vi "solar_voy_def Variant Get TCP.vi"(8 "error in (no error)":errorcluster, 11 "Variant":variant) -> (0 "error out":errorcluster, 2 "LabVIEW Flattened Value":string[](array[string]), 3 "LabVIEW Values":variant[](array[variant]))   [LabVIEW 2018]
doc: "This unpacks a variant into an array of variants. Paths are converted into strings."
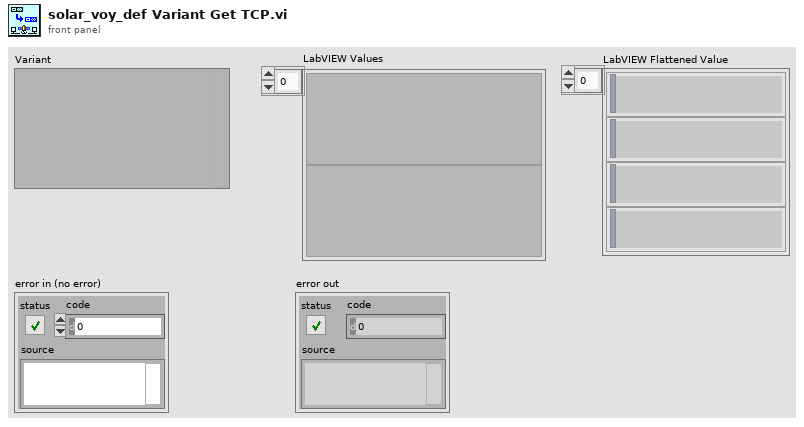
[diagram p1: front panel]
types:
  T1 = typedef "solar_type Item Type.ctl" = enum16{"NULL", "UNKNOWN", "CLUSTER", "I8", "I16", "I32", "I64", "U8", "U16", "U32", "U64", "U8_ENUM", "U16_ENUM", "U32_ENUM", "SGL", "DBL", "BOOLEAN", "STRING", "PATH", "VISA", "TAG", "TIME", "I8_1D", "I16_1D", "I32_1D", "I64_1D", "U8_1D", "U16_1D", "U32_1D", "U64_1D", "U8_ENUM_1D", "U16_ENUM_1D", "U32_ENUM_1D", "SGL_1D", "DBL_1D", "BOOLEAN_1D", "STRING_1D", "PATH_1D", "VISA_1D", "TAG_1D", "TIME_1D", "I8_2D", "I16_2D", "I32_2D", "I64_2D", "U8_2D", "U16_2D", "U32_2D", "U64_2D", "U8_ENUM_2D", "U16_ENUM_2D", "U32_ENUM_2D", "SGL_2D", "DBL_2D", "BOOLEAN_2D", "STRING_2D", "PATH_2D", "VISA_2D", "TAG_2D", "TIME_2D"}
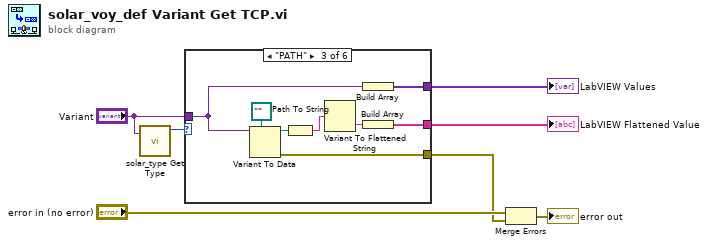
[diagram p0: block diagram]
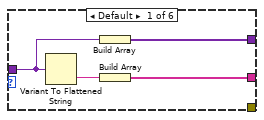
[diagram p2: hidden frame]
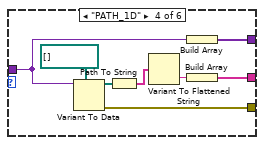
[diagram p4: hidden frame]
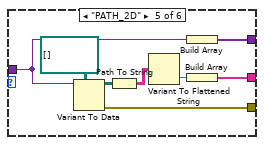
[diagram p5: hidden frame]
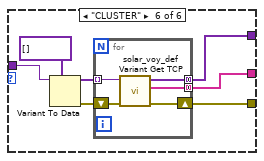
[diagram p6: hidden frame]
diagram:
  n1 = call "solar_type Get Type.vi"("Variant"="Variant") -> ("Type"=w2:T1)  [unwired: 4 in, 2 out]
  n2 = case shown="\"PATH\"" w2 {
    tunnel: "Variant" -> [w9 _ w13 w21 w29 w42]
    tunnel: [w10 _ w14 w22 w30 w39] -> w7
    tunnel: [_ _ w19 w27 w35 w37] -> w5
    tunnel: [w8 _ w12 w20 w28 w36] -> w1
    frame Default {
      n3 = Variant To Flattened String(Variant=w9) -> (data string=w11:string)  [unwired: 1 out]
      n4 = Build Array(w9) -> (w8:variant[])
      n5 = Build Array(w11) -> (w10:string[])
    }
    frame "NULL" {
    }
    frame "PATH" {
      n6 = Variant To Data(type=path "", Variant=w13) -> (data=w17:path, error out=w19:errorcluster)  [unwired: 1 in]
      n7 = Path To String(path=w17) -> (string=w16:string)
      n8 = Variant To Flattened String(Variant=w16) -> (data string=w15:string)  [unwired: 1 out]
      n9 = Build Array(w13) -> (w12:variant[])
      n10 = Build Array(w15) -> (w14:string[])
    }
    frame "PATH_1D" {
      n11 = Variant To Data(type=path[] [], Variant=w21) -> (data=w25:path[], error out=w27:errorcluster)  [unwired: 1 in]
      n12 = Path To String(path=w25) -> (string=w24:string[])
      n13 = Variant To Flattened String(Variant=w24) -> (data string=w23:string)  [unwired: 1 out]
      n14 = Build Array(w21) -> (w20:variant[])
      n15 = Build Array(w23) -> (w22:string[])
    }
    frame "PATH_2D" {
      n16 = Variant To Data(type=path[][] [], Variant=w29) -> (data=w33:path[][], error out=w35:errorcluster)  [unwired: 1 in]
      n17 = Path To String(path=w33) -> (string=w32:string[][])
      n18 = Variant To Flattened String(Variant=w32) -> (data string=w31:string)  [unwired: 1 out]
      n19 = Build Array(w29) -> (w28:variant[])
      n20 = Build Array(w31) -> (w30:string[])
    }
    frame "CLUSTER" {
      n21 = Variant To Data(type=variant[] [], Variant=w42) -> (data=w40:variant[], error out=w38:errorcluster)  [unwired: 1 in]
      n22 = for {
        tunnel: w40 -> [w46] mode=indexing
        tunnel: [w44] -> w39 mode=concatenating
        shift-right: [w45] -> w37
        shift-left: w38 -> [w47]
        tunnel: [w43] -> w36 mode=concatenating
        n23 = call "solar_voy_def Variant Get TCP.vi"("error in (no error)"=w47, "Variant"=w46) -> ("error out"=w45:errorcluster, "LabVIEW Flattened Value"=w44:string[], "LabVIEW Values"=w43:variant[])  [unwired: 7 in]
      }
    }
  }
  "LabVIEW Flattened Value" <- w7
  "LabVIEW Values" <- w1
  n24 = Merge Errors("error in (no error)", w5) -> (→"error out":errorcluster)
